vi "main.vi"() -> ()   [LabVIEW 2015]
uses:
  Stany_enum.ctl
  <vilib>/DAQmx/write.llb/DAQmx Write (Analog Wfm 1Chan NSamp).vi
  <vilib>/DAQmx/read.llb/DAQmx Read (Analog 1D DBL 1Chan NSamp).vi
  <vilib>/DAQmx/create/channels.llb/DAQmx Create Channel (AO-Voltage-Basic).vi
  <vilib>/DAQmx/configure/timing.llb/DAQmx Timing (Use Waveform).vi
  <vilib>/DAQmx/miscellaneous.llb/DAQmx Fill In Error Info.vi
  <vilib>/DAQmx/create/channels.llb/DAQmx Create Channel (AI-Voltage-Basic).vi
  <vilib>/DAQmx/configure/timing.llb/DAQmx Timing (Sample Clock).vi
  <resource>/objmgr/daqmx.rc
panel:
  in  "Sterowanie\naplikacją":cluster{"Start pomiaru":bool, "Stop":bool}
  out "Ostatni błąd":errorcluster
  in  "Ustawienia\npomiaru":T1={"Kanal pomiaru"="", "Czestotliwosc pomiaru"=1000.0, "Liczba probek na kanal pomiarowy"=1000} {"Czestotliwosc pomiaru" format="%0.2f"}
  in  "Ustawienia\ngeneratora":T2={"Kanal generatora"="", "Ksztalt sygnalu"=enum."Sine Wave", "RegenMode"=10097} {"RegenMode" items=["Allow Regeneration"=10097, "Do Not Allow Regeneration"=10158]}
  out "Generowany sygnal":waveform(dbl)(graph)
  out "Pomiar":dbl[](graph)
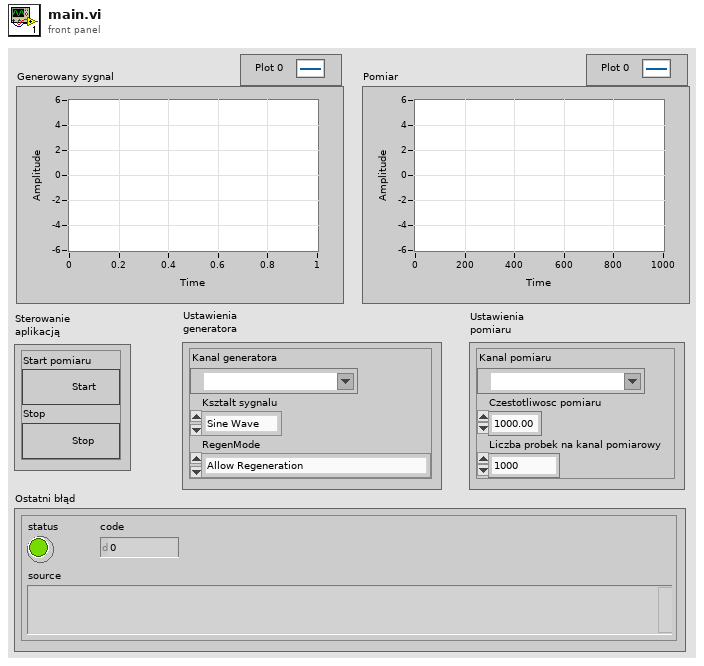
[diagram p1: front panel]
types:
  T1 = cluster{"Kanal pomiaru":tag, "Czestotliwosc pomiaru":dbl, "Liczba probek na kanal pomiarowy":i32}
  T2 = cluster{"Kanal generatora":tag, "Ksztalt sygnalu":enum16{"Sine Wave", "Triangle Wave", "Square Wave", "Sawtooth Wave"}, "RegenMode":i32}
  T3 = typedef "Stany_enum.ctl" = enum16{"Sprawdz czy STOP", "Czekaj na START", "Init", "Pracuj", "STOP", "Blad"}
  T4 = cluster{"RegenMode":refnum<vi>, "Ksztalt sygnalu":refnum<vi>, "Liczba probek na kanal pomiarowy":refnum<vi>, "Czestotliwosc pomiaru":refnum<vi>, "Kanal pomiaru":refnum<vi>, "Kanal generatora":refnum<vi>}
  T5 = enum8{"Enabled", "Disabled", "Disabled and Grayed Out"}
  T6 = enum16{"Sine Wave", "Triangle Wave", "Square Wave", "Sawtooth Wave"}
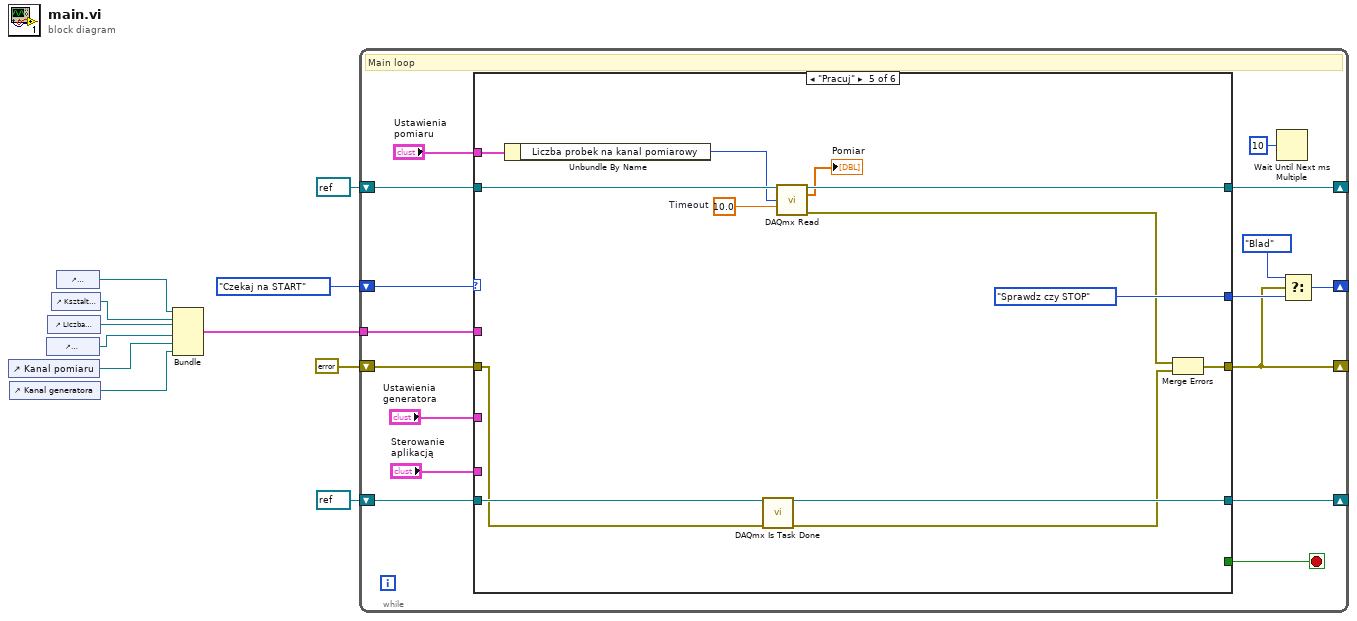
[diagram p0: block diagram]
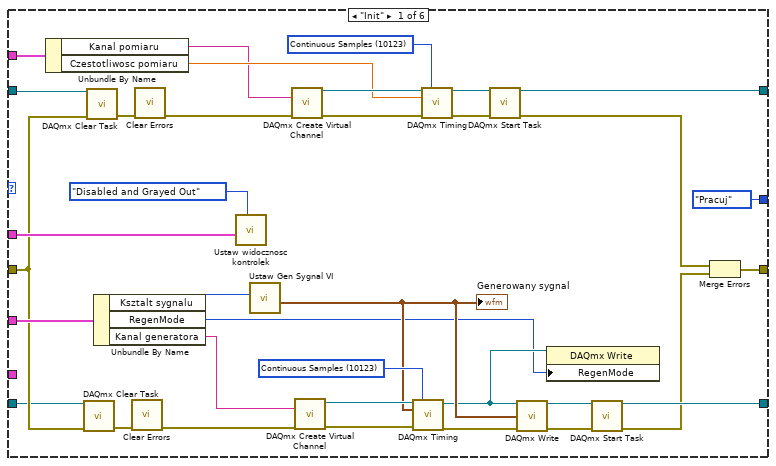
[diagram p2: hidden frame]
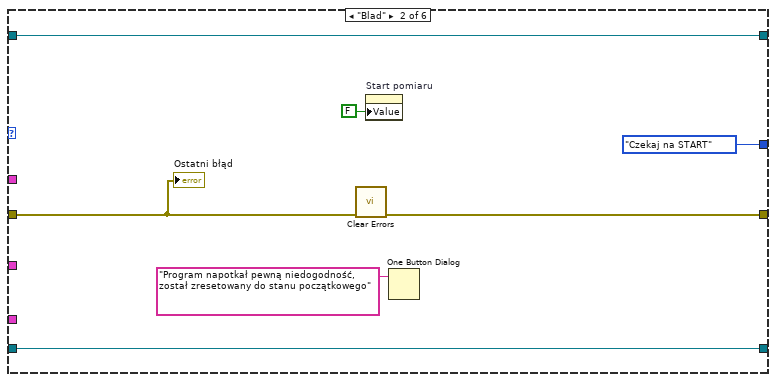
[diagram p3: hidden frame]
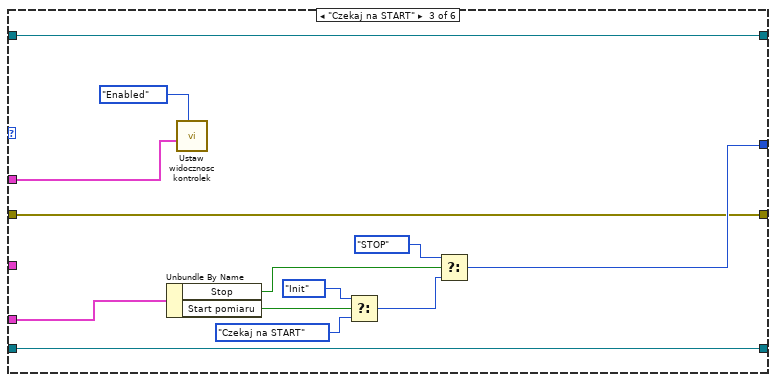
[diagram p4: hidden frame]
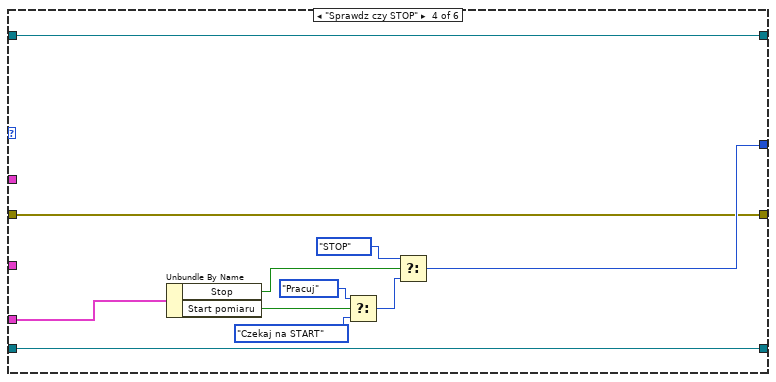
[diagram p5: hidden frame]
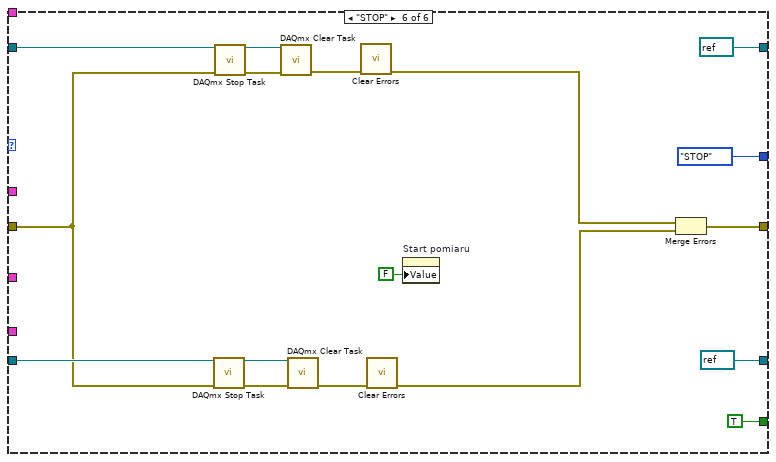
[diagram p6: hidden frame]
diagram:
  n1 = control-ref of="Kanal pomiaru"() -> (w3:refnum<vi>)
  n2 = control-ref of="Kanal generatora"() -> (w2:refnum<vi>)
  n3 = control-ref of="Czestotliwosc pomiaru"() -> (w4:refnum<vi>)
  n4 = control-ref of="Liczba probek na kanal pomiarowy"() -> (w5:refnum<vi>)
  n5 = control-ref of="Ksztalt sygnalu"() -> (w6:refnum<vi>)
  n6 = control-ref of="RegenMode"() -> (w7:refnum<vi>)
  n7 = Bundle("RegenMode"=w7, "Ksztalt sygnalu"=w6, "Liczba probek na kanal pomiarowy"=w5, "Czestotliwosc pomiaru"=w4, "Kanal pomiaru"=w3, "Kanal generatora"=w2) -> (w1:T4)  [unwired: 1 in]
  n8 = while {
    shift-right: [w26] -> _
    shift-left: refnum<k21> refnum ("task out") -> [w24]
    shift-right: [w25] -> _
    shift-left: refnum<k21> refnum ("task out") -> [w23]
    shift-right: [w17] -> _
    shift-left: Stany_enum."Czekaj na START" -> [w27]
    shift-right: [w18] -> _
    shift-left: errorcluster {"status"=FALSE, "code"=0, "source"=""} ("error out") -> [w20]
    tunnel: w1 -> [w12]
    stop <- w22 stop-if-true
    # "Main loop"
    n9 = case shown="\"Pracuj\"" w27 {
      tunnel: [w52 w68 w77 w84 w105 refnum<k21> refnum ("task out")] -> w26
      tunnel: [w51 w69 w78 w89 w103 refnum<k21> refnum ("task out")] -> w25
      tunnel: w24 -> [w30 w68 w77 w84 w106 w117]
      tunnel: w23 -> [w28 w69 w78 w89 w104 w114]
      tunnel: [Stany_enum."Pracuj" Stany_enum."Czekaj na START" w73 w85 Stany_enum."Sprawdz czy STOP" Stany_enum."STOP"] -> w19
      tunnel: [_ _ _ _ _ TRUE] -> w22
      tunnel: "Sterowanie\naplikacją" -> [_ _ w82 w93 _ _]
      tunnel: [w43 w67 w72 w83 w98 w109] -> w18
      tunnel: w20 -> [w29 w63 w72 w83 w99 w110]
      tunnel: "Ustawienia\ngeneratora" -> [w41 _ _ _ _ _]
      tunnel: "Ustawienia\npomiaru" -> [w40 _ _ _ w95 _]
      tunnel: w12 -> [w31 _ w71 _ _ _]
      frame "Init" {
        w54 = 10123 items=["Finite Samples"=10178, "Continuous Samples"=10123, "Hardware Timed Single Point"=12522] ("sample mode")
        w60 = 10123 items=["Finite Samples"=10178, "Continuous Samples"=10123, "Hardware Timed Single Point"=12522] ("sample mode")
        n10 = Unbundle By Name(w40) -> ("Kanal pomiaru"=w38:tag, "Czestotliwosc pomiaru"=w39:dbl)
        n11 = call <vilib>:"DAQmx Clear Task.vi"("task in"=w28, "error in"=w29) -> ("error out"=w47:errorcluster)  [unwired: 13 in]
        n12 = call <vilib>:"DAQmx Clear Task.vi"("task in"=w30, "error in"=w29) -> ("error out"=w49:errorcluster)  [unwired: 13 in]
        n13 = Unbundle By Name(w41) -> ("Ksztalt sygnalu"=w34:T6, "RegenMode"=w33:i32, "Kanal generatora"=w37:tag)
        n14 = call <vilib>:"Clear Errors.vi"("error in (no error)"=w47) -> ("error out"=w46:errorcluster)  [unwired: 5 in, 1 out]
        n15 = call <vilib>:"Clear Errors.vi"("error in (no error)"=w49) -> ("error out"=w48:errorcluster)  [unwired: 5 in, 1 out]
        n16 = call "Ustaw widocznosc kontrolek.vi"("Disabled/Enabled"=T5."Disabled and Grayed Out" ("Disabled"), "Klaster referencji"=w31) -> ()  [unwired: 10 in]
        n17 = call "Ustaw Gen Sygnal VI.vi"("Ksztalt sygnalu"=w34) -> ("generowany sygnal"=w42:waveform(dbl))  [unwired: 10 in]
        "Generowany sygnal" <- w42
        n18 = call-poly <vilib>:"DAQmx Create Virtual Channel.vi"("physical channels"=w38, "error in"=w48) -> ("task out"=w61:refnum<k21>, "error out"=w62:errorcluster)  [unwired: 12 in]
        n19 = call-poly <vilib>:"DAQmx Create Virtual Channel.vi"("physical channels"=w37, "error in"=w46) -> ("task out"=w53:refnum<k21>, "error out"=w55:errorcluster)  [unwired: 12 in]
        n20 = call-poly <vilib>:"DAQmx Timing.vi"("task/channels in"=w53, "sample mode"=w54, "waveform"=w42, "error in"=w55) -> ("task out"=w35:refnum<k21>, "error out"=w56:errorcluster)  [unwired: 10 in]
        n21 = call-poly <vilib>:"DAQmx Timing.vi"("task/channels in"=w61, "sample mode"=w60, "rate"=w39, "error in"=w62) -> ("task out"=w36:refnum<k21>, "error out"=w59:errorcluster)  [unwired: 10 in]
        n22 = call <vilib>:"DAQmx Start Task.vi"("task/channels in"=w36, "error in"=w59) -> ("task out"=w52:refnum<k21>, "error out"=w45:errorcluster)  [unwired: 12 in]
        n23 = call-poly <vilib>:"DAQmx Write.vi"("task/channels in"=w35, "data"=w42, "error in"=w56) -> ("task out"=w58:refnum<k21>, "error out"=w57:errorcluster)  [unwired: 10 in, 1 out]
        n24 = property class="DAQmx Write"(reference=w35, "RegenMode"=w33) -> ()  [unwired: 1 in, 2 out]
        n25 = call <vilib>:"DAQmx Start Task.vi"("task/channels in"=w58, "error in"=w57) -> ("task out"=w51:refnum<k21>, "error out"=w44:errorcluster)  [unwired: 12 in]
        n26 = Merge Errors(w45, w44) -> (w43:errorcluster)
      }
      frame "Blad" {
        n27 = call <vilib>:"Clear Errors.vi"("error in (no error)"=w63) -> ("error out"=w67:errorcluster)  [unwired: 5 in, 1 out]
        n28 = property on="Start pomiaru" class="Bool (strict)"("Value"=FALSE) -> ()  [unwired: 2 in, 2 out]
        n29 = One Button Dialog(message="Program napotkał pewną niedogodność, został zresetowany do stanu początkowego") -> ()  [unwired: 1 in, 1 out]
        "Ostatni błąd" <- w63
      }
      frame "Czekaj na START" {
        n30 = Unbundle By Name(w82) -> ("Stop"=w76:bool, "Start pomiaru"=w81:bool)
        n31 = call "Ustaw widocznosc kontrolek.vi"("Disabled/Enabled"=T5."Enabled", "Klaster referencji"=w71) -> ()  [unwired: 10 in]
        n32 = Select(t=Stany_enum."Init", s=w81, f=Stany_enum."Czekaj na START") -> (s? t:f=w75:T3)
        n33 = Select(t=Stany_enum."STOP", s=w76, f=w75) -> (s? t:f=w73:T3)
      }
      frame "Sprawdz czy STOP" {
        n34 = Unbundle By Name(w93) -> ("Stop"=w88:bool, "Start pomiaru"=w92:bool)
        n35 = Select(t=Stany_enum."Pracuj", s=w92, f=Stany_enum."Czekaj na START") -> (s? t:f=w86:T3)
        n36 = Select(t=Stany_enum."STOP", s=w88, f=w86) -> (s? t:f=w85:T3)
      }
      frame "Pracuj" {
        w102 = 10.0  # Timeout
        n37 = Unbundle By Name(w95) -> ("Liczba probek na kanal pomiarowy"=w94:i32)
        n38 = call <vilib>:"DAQmx Is Task Done.vi"("task/channels in"=w104, "error in"=w99) -> ("task out"=w103:refnum<k21>, "error out"=w96:errorcluster)  [unwired: 11 in, 1 out]
        n39 = call-poly <vilib>:"DAQmx Read.vi"("task/channels in"=w106, "number of samples per channel"=w94, "timeout"=w102) -> ("task out"=w105:refnum<k21>, "data"=→"Pomiar":dbl[], "error out"=w97:errorcluster)  [unwired: 10 in]
        n40 = Merge Errors(w97, w96) -> (w98:errorcluster)
      }
      frame "STOP" {
        n41 = call <vilib>:"DAQmx Stop Task.vi"("task/channels in"=w114, "error in"=w110) -> ("task out"=w115:refnum<k21>, "error out"=w116:errorcluster)  [unwired: 12 in]
        n42 = call <vilib>:"DAQmx Stop Task.vi"("task/channels in"=w117, "error in"=w110) -> ("task out"=w119:refnum<k21>, "error out"=w118:errorcluster)  [unwired: 12 in]
        n43 = call <vilib>:"DAQmx Clear Task.vi"("task in"=w119, "error in"=w118) -> ("error out"=w112:errorcluster)  [unwired: 13 in]
        n44 = call <vilib>:"DAQmx Clear Task.vi"("task in"=w115, "error in"=w116) -> ("error out"=w111:errorcluster)  [unwired: 13 in]
        n45 = call <vilib>:"Clear Errors.vi"("error in (no error)"=w112) -> ("error out"=w108:errorcluster)  [unwired: 5 in, 1 out]
        n46 = call <vilib>:"Clear Errors.vi"("error in (no error)"=w111) -> ("error out"=w107:errorcluster)  [unwired: 5 in, 1 out]
        n47 = property on="Start pomiaru" class="Bool (strict)"("Value"=FALSE ("Start pomiaru")) -> ()  [unwired: 2 in, 2 out]
        n48 = Merge Errors(w108, w107) -> (w109:errorcluster)
      }
    }
    n49 = Wait Until Next ms Multiple(millisecond multiple=u32 10) -> ()  [unwired: 1 out]
    n50 = Select(t=Stany_enum."Blad", s=w18, f=w19) -> (s? t:f=w17:T3)
  }
